vi "SSL_CTX_load_certificate.vi"(8 "error in (no error)":errorcluster, 9 "cert path":T1, 10 "CTX":i32, 11 "path in":path) -> (0 "error out":errorcluster, 2 "CTX":i32, 3 "path out":path)   [LabVIEW 2016, in "AWS_IoT.lvlib"]
doc: "Load client cert, client key, and CA file into SSL_CTX\n\nMIT License\n\nCopyright (c) 2016 Indie-Energy\n\nPermission is hereby granted, free of charge, to any person obtaining a copy\nof this software and associated documentation files (the \"Software\"), to deal\nin the Software without restriction, including without limitation the rights\nto use, copy, modify, merge, publish, distribute, sublicense, and/or sell\ncopies of the Software, and to permit persons to whom the Software is\nfurnished to do so, subject to the following conditions:\n\nThe above copyright notice and this permission notice shall be included in all\ncopies or substantial portions of the Software.\n\nTHE SOFTWARE IS PROVIDED \"AS IS\", WITHOUT WARRANTY OF ANY KIND, EXPRESS OR\nIMPLIED, INCLUDING BUT NOT LIMITED TO THE WARRANTIES OF MERCHANTABILITY,\nFITNESS FOR A PARTICULAR PURPOSE AND NONINFRINGEMENT. IN NO EVENT SHALL THE\nAUTHORS OR COPYRIGHT HOLDERS BE LIABLE FOR ANY CLAIM, DAMAGES OR OTHER\nLIABILITY, WHETHER IN AN ACTION OF CONTRACT, TORT OR OTHERWISE, ARISING FROM,\nOUT OF OR IN CONNECTION WITH THE SOFTWARE OR THE USE OR OTHER DEALINGS IN THE\nSOFTWARE."
uses:
  AWS_IoT.lvlib
  Controls/certs.ctl
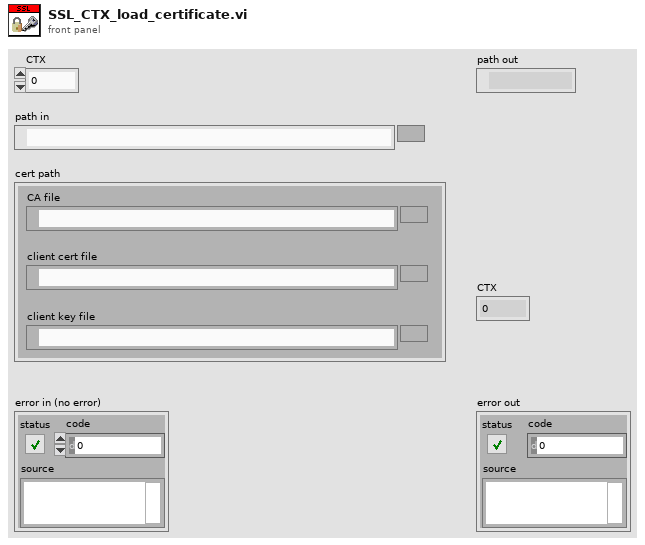
[diagram p1: front panel]
types:
  T1 = typedef "AWS_IoT.lvlib/certs.ctl" = cluster{"client cert file":path, "CA file":path, "client key file":path}
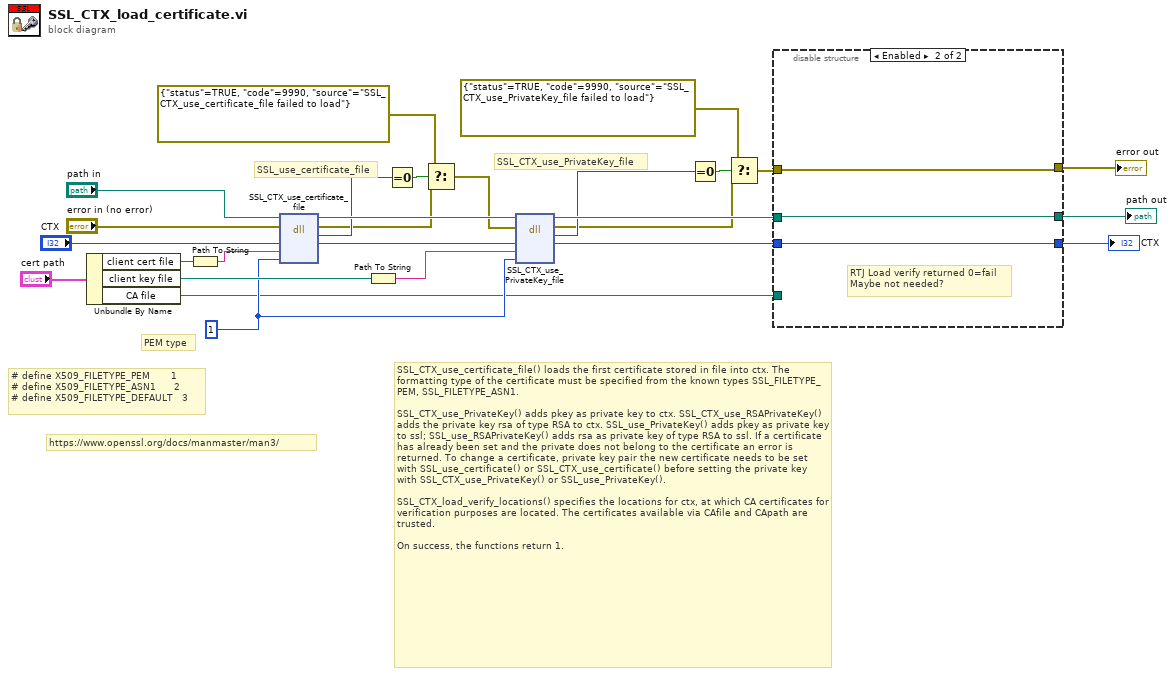
[diagram p0: block diagram]
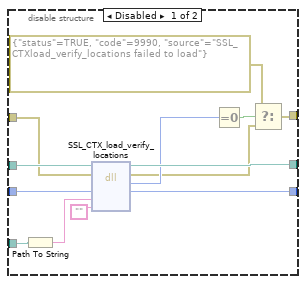
[diagram p2: hidden frame]
diagram:
  w22 = 1 ("type")
  # "https://www.openssl.org/docs/manmaster/man3/"
  # "SSL_CTX_use_certificate_file() loads the first certificate stored in file into ctx. The formatting type of the certificate must be specified from the known types SSL_FILETYPE_PEM, SSL_FILETYPE_ASN1.\n\nSSL_CTX_use_PrivateKey() adds pkey as private key to ctx. SSL_CTX_use_RSAPrivateKey() adds the private key rsa of type RSA to ctx. SSL_use_PrivateKey() adds pkey as private key to ssl; SSL_use_RSAPrivateKey() adds rsa as private key of type RSA to ssl. If a certificate has already been set and the private does not belong to the certificate an error is returned. To change a certificate, private key pair the new certificate needs to be set with SSL_use_certificate() or SSL_CTX_use_certificate() before setting the private key with SSL_CTX_use_PrivateKey() or SSL_use_PrivateKey().\n\nSSL_CTX_load_verify_locations() specifies the locations for ctx, at which CA certificates for verification purposes are located. The certificates available via CAfile and CApath are trusted.\n\nOn success, the functions return 1."
  # "# define X509_FILETYPE_PEM       1\n# define X509_FILETYPE_ASN1      2\n# define X509_FILETYPE_DEFAULT   3"
  # "SSL_CTX_use_PrivateKey_file"
  # "PEM type"
  # "SSL_use_certificate_file"
  n1 = Unbundle By Name("cert path") -> ("client cert file"=w26:path, "client key file"=w27:path, "CA file"=w12:path)
  n2 = Path To String(path=w26) -> (string=w21:string)
  n3 = dll-call lib="NIssleay32.*" fn="SSL_CTX_use_certificate_file"(path in="path in", error in="error in (no error)", "CTX"="CTX", "keyfile"=w21, "type"=w22) -> (path out=w17:path, error out=w8:errorcluster, "return type"=w11:i32, "CTX"=w19:i32)  [unwired: 3 in]
  n4 = Path To String(path=w27) -> (string=w15:string)
  n5 = Equal To 0?(x=w11) -> (x = 0?=w10:bool)
  n6 = Select(t=errorcluster {"status"=TRUE, "code"=9990, "source"="SSL_CTX_use_certificate_file failed to load"}, s=w10, f=w8) -> (s? t:f=w7:errorcluster)
  n7 = dll-call lib="NIssleay32.*" fn="SSL_CTX_use_PrivateKey_file"(path in=w17, error in=w7, "CTX"=w19, "keyfile"=w15, "type"=w22) -> (path out=w14:path, error out=w3:errorcluster, "return type"=w4:i32, "CTX"=w13:i32)  [unwired: 3 in]
  n8 = Equal To 0?(x=w4) -> (x = 0?=w5:bool)
  n9 = Select(t=errorcluster {"status"=TRUE, "code"=9990, "source"="SSL_CTX_use_PrivateKey_file failed to load"}, s=w5, f=w3) -> (s? t:f=w2:errorcluster)
  n10 = disable-structure shown="Enabled" {
    disable-tunnel: [w40 w42] -> w24
    disable-tunnel: [w39 w41] -> w23
    disable-tunnel: w14 -> [w38 w42]
    disable-tunnel: w13 -> [w37 w41]
    disable-tunnel: w12 -> [w34 _]
    disable-tunnel: w2 -> [w30 w43]
    disable-tunnel: [w28 w43] -> w1
    frame Disabled {
      n11 = Path To String(path=w34) -> (string=w35:string)
      n12 = dll-call lib="NIssleay32.*" fn="SSL_CTX_load_verify_locations"(path in=w38, error in=w30, "CTX"=w37, "CAfile"=w35, "CApath"="") -> (path out=w40:path, error out=w29:errorcluster, "return type"=w31:i32, "CTX"=w39:i32)  [unwired: 3 in]
      n13 = Equal To 0?(x=w31) -> (x = 0?=w33:bool)
      n14 = Select(t=errorcluster {"status"=TRUE, "code"=9990, "source"="SSL_CTXload_verify_locations failed to load"}, s=w33, f=w29) -> (s? t:f=w28:errorcluster)
    }
    frame Enabled {
      # "RTJ Load verify returned 0=fail\nMaybe not needed?"
    }
  }
  "CTX" <- w23
  "error out" <- w1
  "path out" <- w24
